vi "Array_Over_Threshold.vi"(1 "Threshold":dbl, 2 "Start Array":dbl[](array[numeric])) -> (0 "OUTPUT ARRAY":dbl[](array[numeric]))   [LabVIEW 2020]
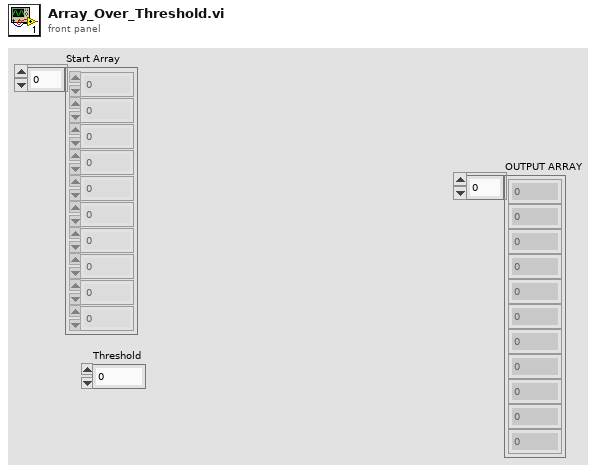
[diagram p1: front panel]
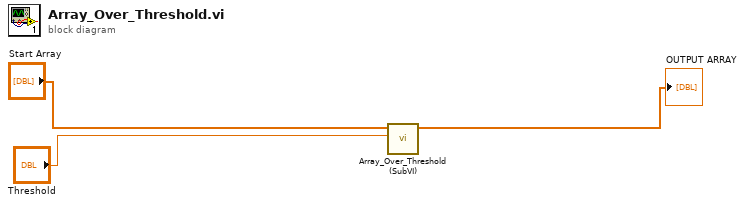
[diagram p0: block diagram]
diagram:
  n1 = call "Array_Over_Threshold (SubVI).vi"("Threshold"="Threshold", "Start Array"="Start Array") -> ("Array"=→"OUTPUT ARRAY":dbl[])  [unwired: 9 in]
